vi "dfd_Group Delay_Initial Guess.vi"(7 "parameter":cluster{"epsilon":dbl, "times":i32}={"epsilon"=1e-05, "times"=300}, 8 "error in (no error)":errorcluster, 10 "Coefficients (array)":T2(array[cluster]), 11 "Design Info":T1={"p"=2, "freq grid"=[], "d"=[], "weight"=[], "Order"=0, "radius"=0.0}) -> (0 "error out":errorcluster, 1 "Error":dbl, 2 "Coefficients (out)":cluster{"r":dbl[], "theta":dbl[], "offset":dbl}, 3 "Design Info (dup)":T1={"p"=2, "freq grid"=[], "d"=[], "weight"=[], "Order"=0, "radius"=0.0})   [LabVIEW 2017, in "NI_DigFilter_Design.lvlib"]
uses:
  <vilib>/addons/Digital Filter Design/NI_DigFilter_Design.lvlib
  <vilib>/addons/Digital Filter Design/_GroupDelay.llb/dfd_Group Delay_Design Info.ctl
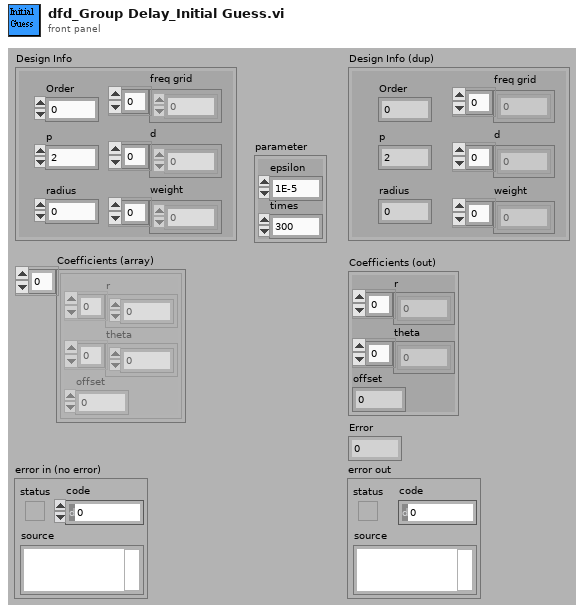
[diagram p1: front panel]
types:
  T1 = typedef "dfd_Group Delay_Design Info.ctl" = cluster{"p":i32, "freq grid":dbl[], "d":dbl[], "weight":dbl[], "Order":i32, "radius":dbl}
  T2 = cluster{"r":dbl[], "theta":dbl[], "offset":dbl}[]
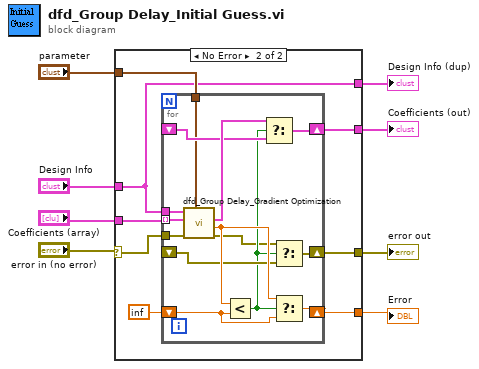
[diagram p0: block diagram]
diagram:
  n1 = case shown="No Error" "error in (no error)" {
    selector: "error in (no error)" -> [w9 w12]
    tunnel: "parameter" -> [_ w17]
    tunnel: "Coefficients (array)" -> [_ w16]
    tunnel: [_ w15] -> w6
    tunnel: [w9 w14] -> w5
    tunnel: [_ w13] -> w4
    tunnel: "Design Info" -> [_ w11]
    tunnel: [_ w11] -> w1
    frame Error {
    }
    frame No Error {
      n2 = for {
        tunnel: w11 -> [w25]
        shift-right: [w28] -> w13
        shift-left: inf -> [w26]
        shift-right: [w31] -> w15
        shift-left: _ -> [w29]
        tunnel: w16 -> [w24] mode=indexing
        tunnel: w12 -> [w23]
        shift-right: [w22] -> w14
        shift-left: _ -> [w21]
        tunnel: w17 -> [w18]
        n3 = call <vilib>:"dfd_Group Delay_Gradient Optimization.vi"("parameter"=w18, "error in (no error)"=w23, "Coefficients (in)"=w24, "Design Info"=w25) -> ("error out"=w19:errorcluster, "Error"=w27:dbl, "Coefficients (out)"=w30:cluster{"r":dbl[], "theta":dbl[], "offset":dbl})  [unwired: 2 in, 3 out]
        n4 = Less?(x=w27, y=w26) -> (x < y?=w20:bool)
        n5 = Select(t=w30, s=w20, f=w29) -> (s? t:f=w31:cluster{"r":dbl[], "theta":dbl[], "offset":dbl})
        n6 = Select(t=w19, s=w20, f=w21) -> (s? t:f=w22:errorcluster)
        n7 = Select(t=w27, s=w20, f=w26) -> (s? t:f=w28:dbl)
      }
    }
  }
  "Coefficients (out)" <- w6
  "error out" <- w5
  "Error" <- w4
  "Design Info (dup)" <- w1
